vi "test_brake_actuation.vi"() -> ()   [LabVIEW 2018]
uses:
  <vilib>/rvi/Emulation/niFpgaGetClockAttributes.vi
  <vilib>/rvi/Emulation/niFpgaSctlEmulationGetInTimedLoop.vi
  <vilib>/rvi/Emulation/niFpgaEmulationReportErrorSimple.vi
  <vilib>/rvi/eio/common/nirviEmuTemplateMethod_errors.vi
  <vilib>/rvi/Emulation/niFpgaCriticalErrorInLSC.vi
  <vilib>/eio/EIONode/EIONode.xnode
panel:
  out "fxp_pressure_22":i32
  out "fxp_pressure_21":i32
  out "fxp_pressure_20":i32
  out "fxp_pressure_19":i32
  out "fxp_pressure_18":i32
  out "fxp_pressure_17":i32
  out "fxp_pressure_16":i32
  out "fxp_pressure_15":i32
  out "fxp_pressure_14":i32
  in  "stop":bool
  out "current_drain_valve_state":bool
  out "current_brake_state":bool
  in  "set_drain_valve":bool
  in  "set_brakes":bool
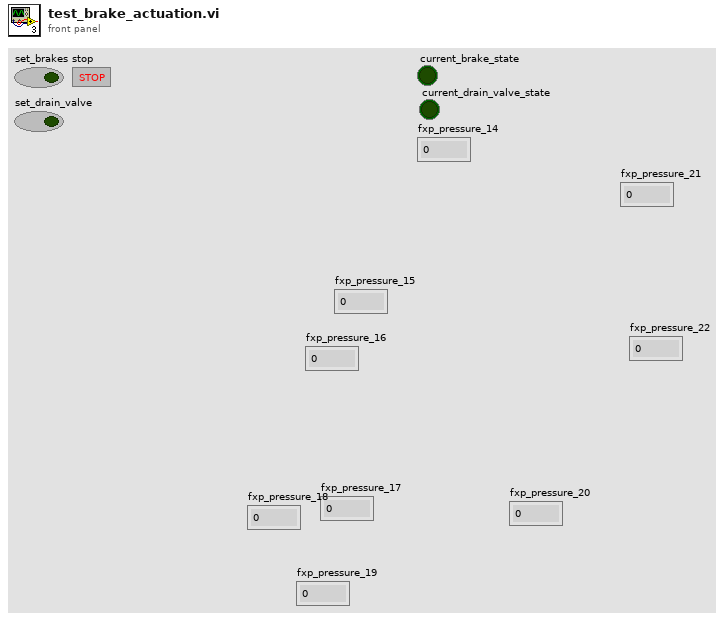
[diagram p1: front panel]
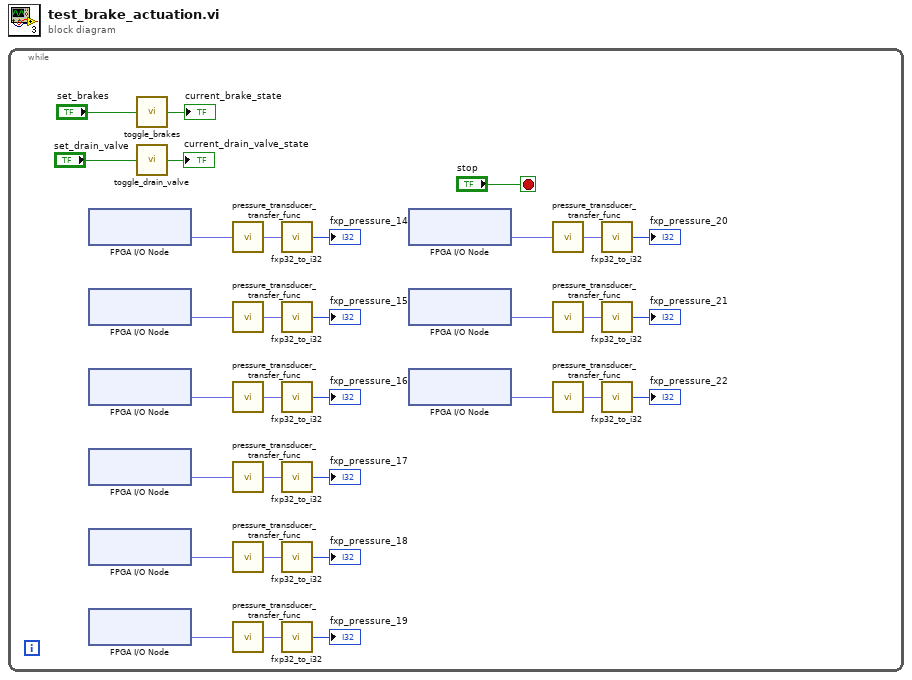
[diagram p0: block diagram]
diagram:
  n1 = while {
    stop <- "stop" stop-if-true
    n2 = xnode "FPGA I/O Node"() -> ("Mod1/AI14"=w28:fxp<+/-,24,5>)  [unwired: 1 in, 1 out]
    n3 = xnode "FPGA I/O Node"() -> ("Mod1/AI15"=w8:fxp<+/-,24,5>)  [unwired: 1 in, 1 out]
    n4 = xnode "FPGA I/O Node"() -> ("Mod1/AI16"=w7:fxp<+/-,24,5>)  [unwired: 1 in, 1 out]
    n5 = xnode "FPGA I/O Node"() -> ("Mod1/AI17"=w6:fxp<+/-,24,5>)  [unwired: 1 in, 1 out]
    n6 = xnode "FPGA I/O Node"() -> ("Mod1/AI18"=w5:fxp<+/-,24,5>)  [unwired: 1 in, 1 out]
    n7 = xnode "FPGA I/O Node"() -> ("Mod1/AI19"=w4:fxp<+/-,24,5>)  [unwired: 1 in, 1 out]
    n8 = call "toggle_brakes.vi"("set_brakes"="set_brakes") -> ("current_brake_state"=→"current_brake_state":bool)
    n9 = call "toggle_drain_valve.vi"("set_drain_valve"="set_drain_valve") -> ("current_drain_valve_state"=→"current_drain_valve_state":bool)
    n10 = call "pressure_transducer_transfer_func.vi"("p_v"=w28) -> ("pressure"=w27:fxp<+/-,32,16>)
    n11 = call "pressure_transducer_transfer_func.vi"("p_v"=w8) -> ("pressure"=w24:fxp<+/-,32,16>)
    n12 = call "pressure_transducer_transfer_func.vi"("p_v"=w7) -> ("pressure"=w22:fxp<+/-,32,16>)
    n13 = call "pressure_transducer_transfer_func.vi"("p_v"=w6) -> ("pressure"=w20:fxp<+/-,32,16>)
    n14 = call "pressure_transducer_transfer_func.vi"("p_v"=w5) -> ("pressure"=w18:fxp<+/-,32,16>)
    n15 = call "pressure_transducer_transfer_func.vi"("p_v"=w4) -> ("pressure"=w16:fxp<+/-,32,16>)
    n16 = call "fxp32_to_i32.vi"("fxp32_16"=w27) -> ("32bit integer"=→"fxp_pressure_14":i32)
    n17 = call "fxp32_to_i32.vi"("fxp32_16"=w24) -> ("32bit integer"=→"fxp_pressure_15":i32)
    n18 = call "fxp32_to_i32.vi"("fxp32_16"=w22) -> ("32bit integer"=→"fxp_pressure_16":i32)
    n19 = call "fxp32_to_i32.vi"("fxp32_16"=w20) -> ("32bit integer"=→"fxp_pressure_17":i32)
    n20 = call "fxp32_to_i32.vi"("fxp32_16"=w18) -> ("32bit integer"=→"fxp_pressure_18":i32)
    n21 = call "fxp32_to_i32.vi"("fxp32_16"=w16) -> ("32bit integer"=→"fxp_pressure_19":i32)
    n22 = xnode "FPGA I/O Node"() -> ("Mod1/AI20"=w3:fxp<+/-,24,5>)  [unwired: 1 in, 1 out]
    n23 = xnode "FPGA I/O Node"() -> ("Mod1/AI21"=w2:fxp<+/-,24,5>)  [unwired: 1 in, 1 out]
    n24 = xnode "FPGA I/O Node"() -> ("Mod1/AI22"=w1:fxp<+/-,24,5>)  [unwired: 1 in, 1 out]
    n25 = call "pressure_transducer_transfer_func.vi"("p_v"=w3) -> ("pressure"=w14:fxp<+/-,32,16>)
    n26 = call "pressure_transducer_transfer_func.vi"("p_v"=w2) -> ("pressure"=w12:fxp<+/-,32,16>)
    n27 = call "pressure_transducer_transfer_func.vi"("p_v"=w1) -> ("pressure"=w10:fxp<+/-,32,16>)
    n28 = call "fxp32_to_i32.vi"("fxp32_16"=w14) -> ("32bit integer"=→"fxp_pressure_20":i32)
    n29 = call "fxp32_to_i32.vi"("fxp32_16"=w12) -> ("32bit integer"=→"fxp_pressure_21":i32)
    n30 = call "fxp32_to_i32.vi"("fxp32_16"=w10) -> ("32bit integer"=→"fxp_pressure_22":i32)
  }
